vi "Get Digital Vars.vi"(0 "Common alarm handling(F)":bool, 7 "Tool":bool, 11 "error in (no error)":errorcluster) -> (4 "Catagorised  Stsaus":T1[](array[typedef]), 6 "Values":T4[](array[typedef]), 8 "Analog Vars":T5[](array[typedef]), 10 "Any Alarm":bool, 13 "Primary Action":T3, 14 "Alarms":bool[](array[boolean]), 15 "error out":errorcluster)   [LabVIEW 2011]
uses:
  Digital GUI/Digital Display cluster.ctl
  Digital GUI/Digital Disp small indicator.ctl
  GUI/Status indicator white.ctl
  Status Digitalish.ctl
  Action List.ctl
  Catagorised alarm state.ctl
  GUI/Status Indikator Helper.ctl
  Common/Variable List Common Digital.ctl
  Common/Variable List Common Analog.ctl
  Action Analog Handler.ctl
  <vilib>/Utility/VariantDataType/GetNumericInfo.vi
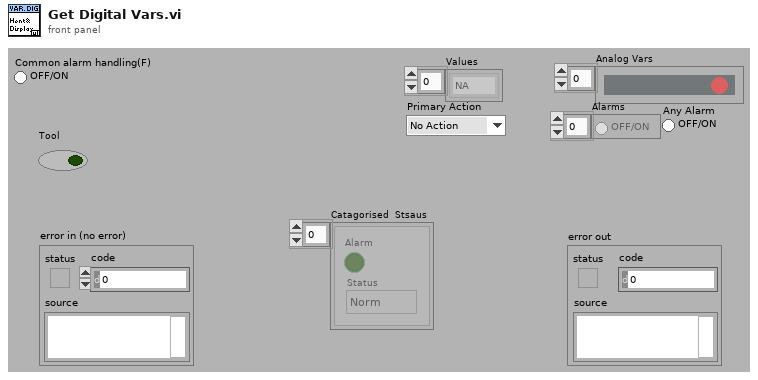
[diagram p1: front panel]
types:
  T1 = typedef "Catagorised alarm state.ctl" = cluster{"Alarm":bool, "Status":T2}
  T2 = typedef "Status Indikator Helper.ctl" = enum16{"Norm", "L", "H", "LL", "HH", "Value", "Technical"}
  T3 = typedef "Action List.ctl" = enum16{"No Action", "Stop Motor", "Turn Off HV"}
  T4 = typedef "Status Digitalish.ctl" = enum16{"NA", "False", "True"}
  T5 = typedef "Digital Display cluster.ctl" = cluster{"ON/OFF TEXT":string, "Val":T6, "Status":T7}
  T6 = typedef "Digital Disp small indicator.ctl" = u16
  T7 = typedef "Status indicator white.ctl" = u16
  T8 = typedef "Variable List Common Digital.ctl" = enum16{"PCP Connected", "PCP PC Control", "HV PSU connected", "HV PSU HV Active", "Modem Connected", "Tool Connected", "CanBus interface"}
  T9 = typedef "Variable List Common Analog.ctl" = enum16{"HVPSU Head Voltage", "HVPSU TS Voltage", "HVPSU Current", "PCP Cable Resistance", "Winch Depth", "Winch Line Speed", "Winch Wire Tension"}
  T10 = typedef "Action Analog Handler.ctl" = enum16{"GET value", "GET Single Frequenzy", "GET All Values", "GET Waveform", "Get Numb Var", "SET Value", "START Buffer", "REG Variable", "BUF size(total antal sekund)", "PULS", "Get a Value at time", "Set initial waveform"}
  T11 = typedef "User Setting DigitalChannel.ctl" = cluster{"Responses":cluster{"Technical Error (NA)":T12, "OFF / FALSE":T13, "ON / TRUE":T13}}
  T12 = typedef "Alarm Responce.ctl" = cluster{"Action":T3, "Alarm":bool}
  T13 = typedef "Alarm Responce dig.ctl" = cluster{"Action":T3, "Alarm":bool, "Exclamation":bool}
  T14 = typedef "Fixed Digital Channel Definition.ctl" = cluster{"ID":u16, "Name":string, "NA Text":string, "Off Text":string, "On Text":string, "Maximum upd":T15, "Comment":string, "Help file Name":string, "Help file Section ":string, "Catagory":T16, "In use":bool}
  T15 = typedef "Update frequensies.ctl" = enum16{"2 Hz", "1 Hz", "0.1 Hz"}
  T16 = typedef "Channel catagory Enum.ctl" = enum16{"No Category", "Power", "Temperature", "Pressure"}
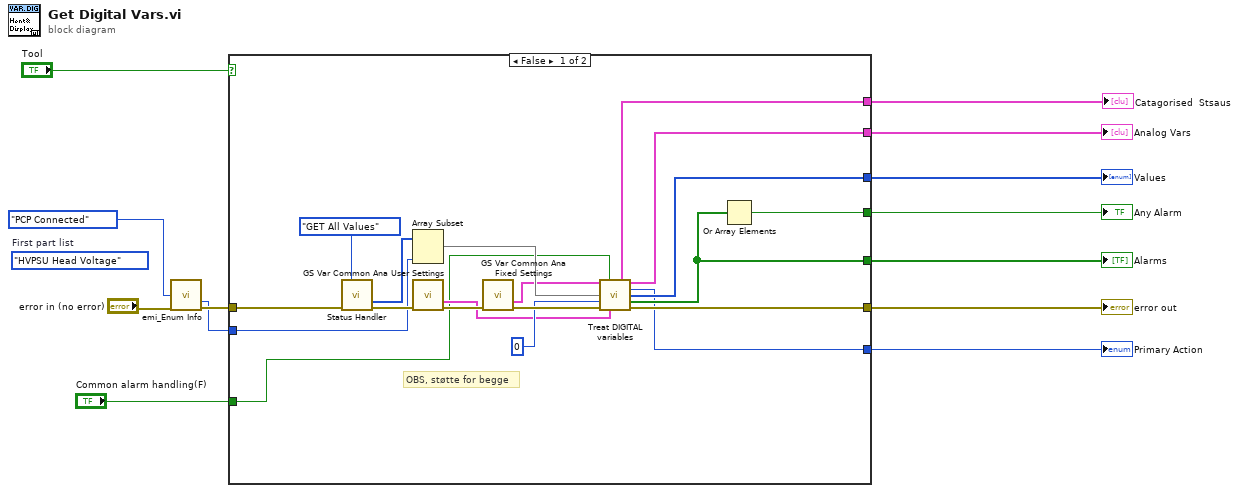
[diagram p0: block diagram]
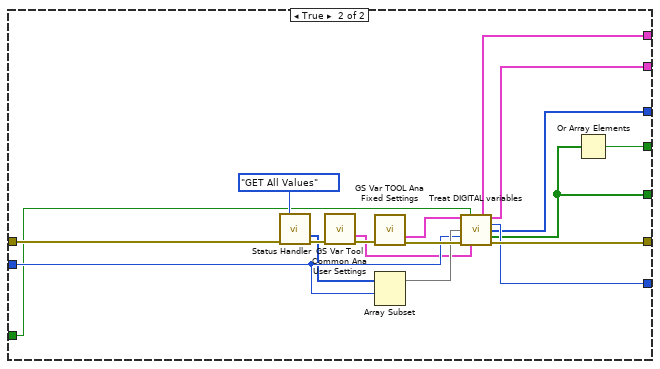
[diagram p2: hidden frame]
diagram:
  (unwired) Variable_List_Common_Analog."HVPSU Head Voltage"  # First part list
  n1 = call "emi_Enum Info.vi"("Enum"=Variable_List_Common_Digital."PCP Connected" ("Action"), "error in (no error)"="error in (no error)") -> ("Numb Elements"=w6:i32, "error out"=w7:errorcluster)  [unwired: 10 in, 2 out]
  n2 = case shown="False" "Tool" {
    tunnel: [w29 w38] -> w13
    tunnel: [w28 w41] -> w12
    tunnel: [w27 w40] -> w11
    tunnel: [w26 w44] -> w10
    tunnel: [w25 w39] -> w9
    tunnel: w7 -> [w24 w45]
    tunnel: w6 -> [w21 w43]
    tunnel: [w20 w42] -> w5
    tunnel: [w18 w37] -> w4
    tunnel: "Common alarm handling(F)" -> [w14 w33]
    frame False {
      # "OBS, støtte for begge"
      n3 = call "Status Handler.vi"("Action"=Action_Analog_Handler."GET All Values" ("Action(GET)"), "error in (no error)"=w24) -> ("Values"=w15:T4[], "error out"=w23:errorcluster)  [unwired: 9 in, 3 out]
      n4 = Array Subset(array=w15, length=w21) -> (w22:T4[])  [unwired: 1 in]
      n5 = call "GS Var Common Ana User Settings.vi"("error in (no error)"=w23) -> ("Common Digital Var User set out"=w17:T11[], "error out"=w30:errorcluster)  [unwired: 12 in, 1 out]
      n6 = call "GS Var Common Ana Fixed Settings.vi"("error in (no error)"=w30) -> ("Common Digital var Fixed"=w16:T14[], "error out"=w32:errorcluster)  [unwired: 12 in, 1 out]
      n7 = call "Treat DIGITAL variables.vi"("Analog Variable info fixed"=w16, "Common alarm handling(F)"=w14, "Status Values"=w22, "Variabel start index"=0, "error In"=w32, "Analog Variable info Settings"=w17) -> ("Categorized  Status"=w18:T1[], "Digital Variable Display"=w29:T5[], "Action"=w20:T3, "Digital status Values"=w25:T4[], "Alarms"=w28:bool[], "error out"=w26:errorcluster)  [unwired: 3 in, 1 out]
      n8 = Or Array Elements(Boolean array=w28) -> (logical OR=w27:bool)
    }
    frame True {
      n9 = call "Status Handler.vi"("Action"=Action_Analog_Handler."GET All Values" ("Action(GET)"), "error in (no error)"=w45) -> ("Values"=w34:T4[], "error out"=w49:errorcluster)  [unwired: 9 in, 3 out]
      n10 = call "GS Var Tool Common Ana User Settings.vi"("error in (no error)"=w49) -> ("Tool digital var User settigns out"=w36:T11[], "error out"=w48:errorcluster)  [unwired: 12 in, 1 out]
      n11 = call "GS Var TOOL Ana Fixed Settings.vi"("error in (no error)"=w48) -> ("Tool Digital Var Fixed out"=w35:T14[], "error out"=w47:errorcluster)  [unwired: 12 in, 1 out]
      n12 = Array Subset(array=w34, index=w43) -> (w46:T4[])  [unwired: 1 in]
      n13 = call "Treat DIGITAL variables.vi"("Analog Variable info fixed"=w35, "Common alarm handling(F)"=w33, "Status Values"=w46, "Variabel start index"=w43, "error In"=w47, "Analog Variable info Settings"=w36) -> ("Categorized  Status"=w37:T1[], "Digital Variable Display"=w38:T5[], "Action"=w42:T3, "Digital status Values"=w39:T4[], "Alarms"=w41:bool[], "error out"=w44:errorcluster)  [unwired: 3 in, 1 out]
      n14 = Or Array Elements(Boolean array=w41) -> (logical OR=w40:bool)
    }
  }
  "Analog Vars" <- w13
  "Alarms" <- w12
  "Any Alarm" <- w11
  "error out" <- w10
  "Values" <- w9
  "Primary Action" <- w5
  "Catagorised  Stsaus" <- w4
